vi "CSGaussmeter.Zero.vi"(0 "i ref in":refnum<vi>, 11 "error in (no error)":errorcluster) -> (4 "i ref out":refnum<vi>, 15 "error out":errorcluster)   [LabVIEW 2014, in "CSGaussmeter.lvlib"]
doc: "The VI starts the function Zero.\n\n Durch die Funktion Zero wird die Sonde auf 'Null' gesetzt und/oder kleine Felder (z.B. das Erdfeld) unterdrückt. Normalerweise wird dafür die Sonde in die Nullfeldkammer gesteckt."
uses:
  CSGaussmeter.lvlib
  CS_Core/CSObj/CSObj.lvlib
  CSlibraries/UtilityLib/UtilityLib.lvlib
  instr.lib/FH_55/FH 55.lvlib
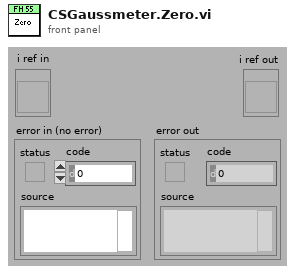
[diagram p1: front panel]
types:
  T1 = typedef "CSGaussmeter.lvlib/CSGaussmeter.i attribute.ctl" = cluster{"Name":string, "VISA Resource Name":refnum<visa-resource-name>, "actValues":cluster{" Limit":bool, "Unit ":T2, "Temp_Unit":T3, "Max":T4, " Filter":bool, " Peak":bool, " Auto_Range":bool, "Range":T5, " Rel":bool, " CTemp":bool, " CField":bool, "AC_DC ":bool, "Set_lower":cluster{"Numeric":dbl, "Cancel Button":bool, "Unit":T6}, "Set_upper":cluster{"Numeric":dbl, "Cancel Button":bool, "Unit":T6}, "Set_Rel":cluster{"Numeric":dbl, "Cancel Button":bool, "Unit":T6}, "Zero":bool, " Local":bool, "Reset":bool, " Init":bool}, "FH 55 Gauss-/Teslameter":T7, "MAX_Value":T8, "MIN_Value":T8, "Rel_Value":T8, "Array ":string[], "LIMU":dbl, " LIML":dbl, "Messwerte 2":string, "Messwerte ":cluster{"Numeric":i32, "OK Button":bool}, "serviceID":cluster{"Current ID":i32, "Unit ID":i32, "Temp ID":i32, "Name ID \n":i32, "Visa ID ":i32}, "setValues ":cluster{" Limit":bool, "Unit ":T2, "Temp_Unit":T3, "Max":T4, " Filter":bool, " Peak":bool, " Auto_Range":bool, "Range":T5, " Rel":bool, " CTemp":bool, " CField":bool, "AC_DC ":bool, "Set_lower":cluster{"Numeric":dbl, "Cancel Button":bool, "Unit":T6}, "Set_upper":cluster{"Numeric":dbl, "Cancel Button":bool, "Unit":T6}, "Set_Rel":cluster{"Numeric":dbl, "Cancel Button":bool, "Unit":T6}, "Zero":bool, " Local":bool, "Reset":bool, " Init":bool}}
  T2 = typedef "FH 55.lvlib/Unit.ctl" = enum16{"T", "G", "A/m"}
  T3 = typedef "FH 55.lvlib/Temp_Unit.ctl" = enum16{"Temp off", "Celsius", "Fahrenheit"}
  T4 = typedef "FH 55.lvlib/Max.ctl" = enum16{"MAX off", "Show MAX", "MAX/MIN"}
  T5 = typedef "FH 55.lvlib/Range.ctl" = enum16{"1", "2", "3", "4", "5", "6", "7"}
  T6 = typedef "FH 55.lvlib/Unit2.ctl" = enum16{"mT", "G", "kA/m"}
  T7 = typedef "FH 55.lvlib/Display.ctl" = cluster{"current value":string, "Limit":string, "Remote":string, "function ":string, "Cluster":cluster{"AC/DC":string, "Auto":string, "Filter":string, "Range":string, "Rel":string, "Peak":string}}
  T8 = typedef "FH 55.lvlib/Value_String.ctl" = cluster{"Numeric":dbl, "String":string}
  T9 = cluster{"VISA Resource Name":refnum<visa-resource-name>}
  T10 = typedef "FH 55.lvlib/VisaCluster.ctl" = cluster{"VISA Resource Name":refnum<visa-resource-name>}
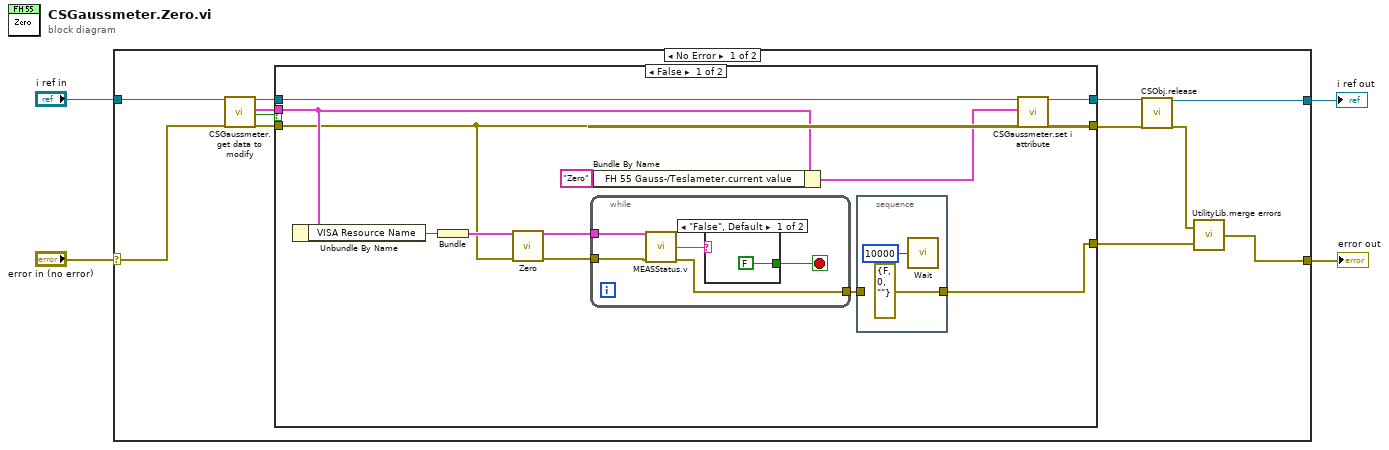
[diagram p0: block diagram]
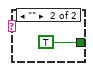
[diagram p2: hidden frame]
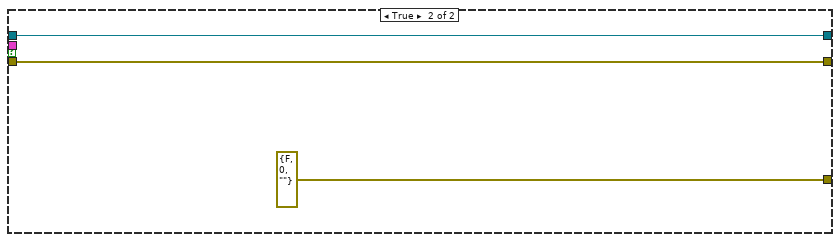
[diagram p3: hidden frame]
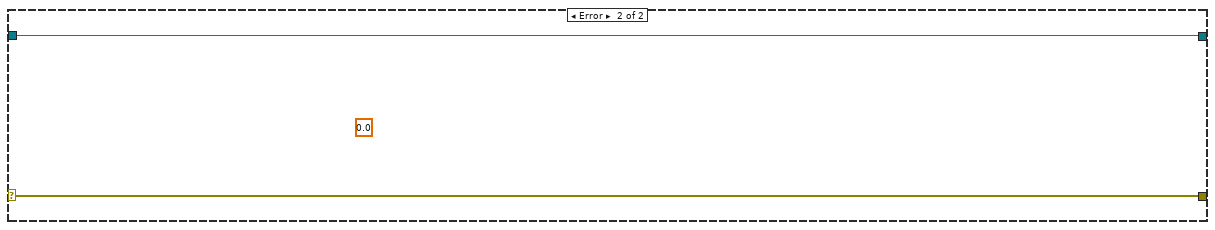
[diagram p4: hidden frame]
diagram:
  n1 = case shown="No Error" "error in (no error)" {
    selector: "error in (no error)" -> [w11 w41]
    tunnel: [w12 w41] -> w1
    tunnel: "i ref in" -> [w10 w42]
    tunnel: [w5 w42] -> w2
    frame No Error {
      n2 = call "CSGaussmeter.get data to modify.vi"("i ref in"=w10, "error in (no error)"=w11) -> ("i ref out"=w9:refnum<vi>, "i attribute"=w8:T1, "timed out"=w7:bool, "error out"=w6:errorcluster)  [unwired: 14 in]
      n3 = case shown="False" w7 {
        tunnel: w9 -> [w26 w39]
        tunnel: w6 -> [w22 w40]
        tunnel: w8 -> [w27 _]
        tunnel: [w22 w40] -> w14
        tunnel: [w24 w39] -> w16
        tunnel: [w17 errorcluster {"status"=FALSE, "code"=0, "source"=""} ("error out")] -> w13
        frame False {
          n4 = Unbundle By Name(w27) -> ("VISA Resource Name"=w28:refnum<visa-resource-name>)
          n5 = Bundle("VISA Resource Name"=w28) -> (w23:T9)  [unwired: 1 in]
          n6 = call "Zero.vi"("VisaCluster"=w23, "error in (no error)"=w22) -> ("VisaCluster"=w19:T10, "error out"=w18:errorcluster)  [unwired: 11 in, 1 out]
          n7 = while {
            tunnel: w19 -> [w35]
            tunnel: w18 -> [w32]
            tunnel: [w31] -> w20
            stop <- w33 stop-if-true
            n8 = call "MEASStatus.v.vi"("VisaCluster"=w35, "error in (no error)"=w32) -> ("Answer"=w34:string, "error out"=w31:errorcluster)  [unwired: 11 in, 1 out]
            n9 = case shown="\"False\", Default" w34 {
              tunnel: [FALSE TRUE] -> w33
              frame "False", Default {
              }
              frame "" {
              }
            }
          }
          n10 = Bundle By Name(cluster=w27, "FH 55 Gauss-/Teslameter.current value"="Zero") -> (w25:T1)
          n11 = stacked-sequence {
            tunnel: w20 -> [_]
            tunnel: [errorcluster {"status"=FALSE, "code"=0, "source"=""} ("error out")] -> w17
            frame #0 {
              n12 = call "Wait.vi"("milliseconds to wait"=u32 10000) -> ()  [unwired: 14 in, 1 out]
            }
          }
          n13 = call "CSGaussmeter.set i attribute.vi"("i ref in"=w26, "i attribute"=w25) -> ("i ref out"=w24:refnum<vi>)  [unwired: 16 in, 1 out]
        }
        frame True {
        }
      }
      n14 = call "CSObj.release.vi"("i ref in"=w16, "error in (no error)"=w14) -> ("i ref out"=w5:refnum<vi>, "error out"=w15:errorcluster)  [unwired: 16 in]
      n15 = call "UtilityLib.merge errors.vi"("error2 (no error)"=w13, "error1 (no error)"=w15) -> ("error out"=w12:errorcluster)
    }
    frame Error {
      (unwired) 0.0 ("Mid Setting [A or T]")
    }
  }
  "i ref out" <- w2
  "error out" <- w1
